vi "CFTS-Get Vital Signs.vi"(9 "timeout ms (500)":i32=500) -> (6 "HR":string, 10 "Temp":string)   [LabVIEW 2020]
panel:
  out "Temp":dbl
  out "HR":dbl
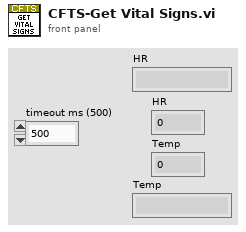
[diagram p1: front panel]
types:
  T1 = enum16{"Standard", "Buffered", "CRLF", "Immediate"}
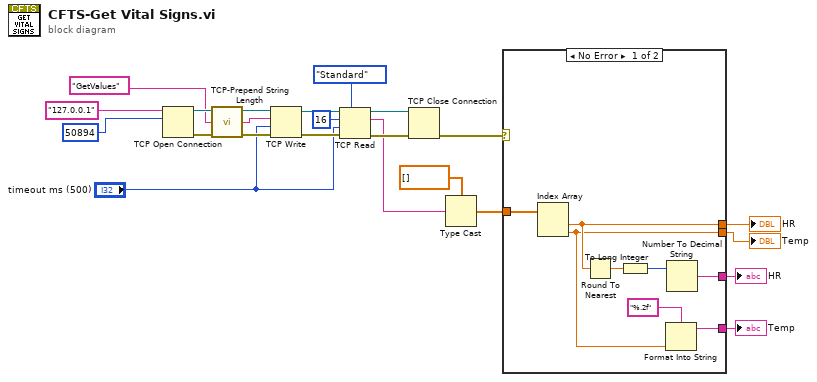
[diagram p0: block diagram]
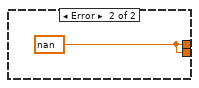
[diagram p2: hidden frame]
diagram:
  n1 = TCP Open Connection(address="127.0.0.1", remote port or service name=50894 ("Port")) -> (connection ID=w21:refnum<k5>, error out=w15:errorcluster)  [unwired: 3 in]
  n2 = call "TCP-Prepend String Length.vi"("Command"="GetValues") -> ("String"=w14:string)  [unwired: 4 in]
  n3 = TCP Write(connection ID=w21, data in=w14, error in (no error)=w15, 9:"timeout ms (500)") -> (connection ID out=w20:refnum<k5>, error out=w16:errorcluster)  [unwired: 1 out]
  n4 = TCP Read(connection ID=w20, bytes to read=16, error in (no error)=w16, 7:T1."Standard" ("mode (standard)"), 9:"timeout ms (500)") -> (connection ID out=w19:refnum<k5>, data out=w8:string, error out=w13:errorcluster)
  n5 = TCP Close Connection(connection ID=w19, error in (no error)=w13) -> (error out=w6:errorcluster)  [unwired: 1 in, 1 out]
  n6 = Type Cast(type=dbl[] [], x=w8) -> (*(type *) &x=w5:dbl[])
  n7 = case shown="No Error" w6 {
    tunnel: w5 -> [w29 _]
    tunnel: [w28 w30] -> w4
    tunnel: [w24 w30] -> w3
    tunnel: [w25 _] -> w2
    tunnel: [w22 _] -> w1
    frame No Error {
      n8 = Index Array(array=w29) -> (element #1=w28:dbl, element #2=w24:dbl)  [unwired: 2 in]
      n9 = Round To Nearest(number=w28) -> (nearest integer value=w27:dbl)
      n10 = To Long Integer(number=w27) -> (32bit integer=w26:i32)
      n11 = Format Into String(format string="%.2f", w24) -> (resulting string=w22:string)  [unwired: 2 in, 1 out]
      n12 = Number To Decimal String(number=w26) -> (decimal integer string=w25:string)  [unwired: 1 in]
    }
    frame Error {
      w30 = nan ("Numeric")
    }
  }
  "HR" <- w4
  "Temp" <- w3
  "HR" <- w2
  "Temp" <- w1
